vi "Colour to RGB.vi"(8 "error in (no error)":errorcluster, 11 "Color":u32(colorbox)) -> (0 "error out":errorcluster, 1 "Blue":u8, 2 "Green":u8, 3 "Red":u8, 5 "Resolved Color":u32 format="%.0x")   [LabVIEW 2018, in "Colour Lab.lvlib"]
uses:
  Colour Lab.lvlib
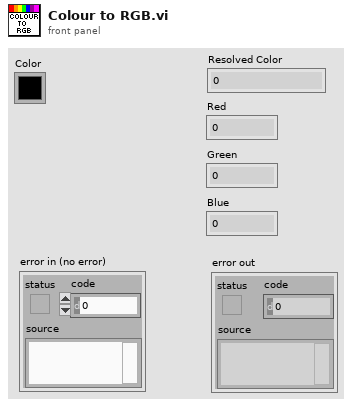
[diagram p1: front panel]
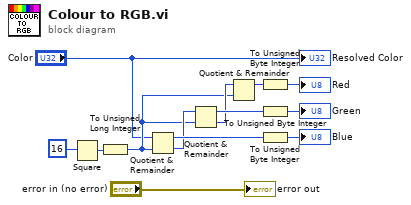
[diagram p0: block diagram]
diagram:
  n1 = Square(x=16) -> (x^2=w8:i32)
  n2 = To Unsigned Long Integer(number=w8) -> (unsigned 32bit integer=w7:u32)
  n3 = Quotient & Remainder(x="Color", y=w7) -> (x-y*floor(x/y)=w12:u32, floor(x/y)=w11:u32)
  n4 = Quotient & Remainder(x=w11, y=w7) -> (x-y*floor(x/y)=w10:u32, floor(x/y)=w9:u32)
  n5 = Quotient & Remainder(x=w9, y=w7) -> (x-y*floor(x/y)=w3:u32)  [unwired: 1 out]
  n6 = To Unsigned Byte Integer(number=w3) -> (unsigned 8bit integer=→"Red":u8)
  n7 = To Unsigned Byte Integer(number=w10) -> (unsigned 8bit integer=→"Green":u8)
  n8 = To Unsigned Byte Integer(number=w12) -> (unsigned 8bit integer=→"Blue":u8)
  "Resolved Color" <- "Color"
  "error out" <- "error in (no error)"
